vi "cRIO AI data2.vi"(0 "I":dbl, 1 "Input cluster":T1, 5 "error in (no error)":errorcluster, 6 "Chan 1":bool, 7 "Scale factor0":dbl, 9 "Scale factor1":dbl, 10 "Chan 2":bool, 11 "Scale factor2":dbl, 12 "Chan 3":bool, 13 "Scale factor3":dbl) -> (14 "Output data":dbl[](array[numeric]), 19 "error out":errorcluster)   [LabVIEW 2020]
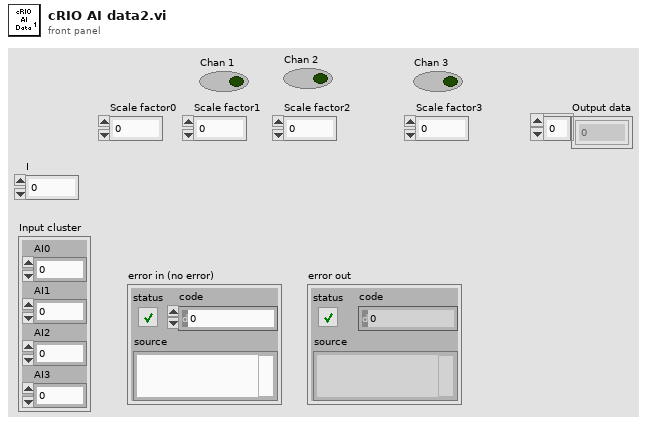
[diagram p1: front panel]
types:
  T1 = cluster{"AI0":dbl, "AI1":dbl, "AI2":dbl, "AI3":dbl}
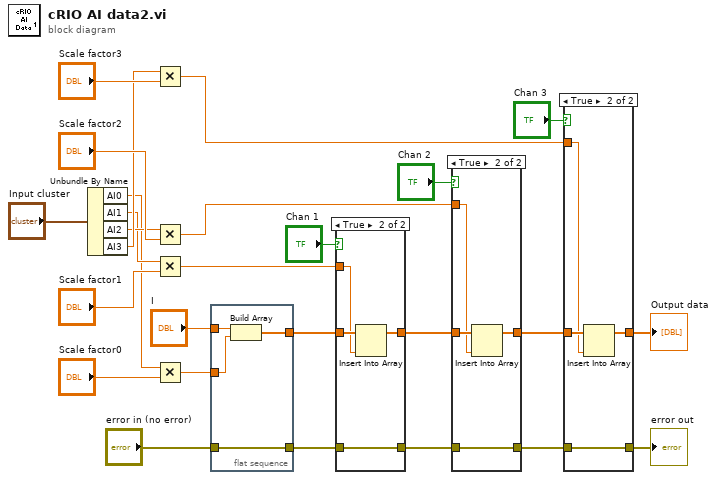
[diagram p0: block diagram]
diagram:
  n1 = Unbundle By Name("Input cluster") -> ("AI0"=w2:dbl, "AI1"=w3:dbl, "AI2"=w4:dbl, "AI3"=w5:dbl)
  n2 = Multiply(x=w5, y="Scale factor3") -> (x*y=w20:dbl)
  n3 = Multiply(x=w4, y="Scale factor2") -> (x*y=w19:dbl)
  n4 = Multiply(x=w3, y="Scale factor1") -> (x*y=w18:dbl)
  n5 = Multiply(x=w2, y="Scale factor0") -> (x*y=w17:dbl)
  n6 = flat-sequence {
    tunnel: "error in (no error)" -> [w30]
    tunnel: [w30] -> w13
    tunnel: w17 -> [w28]
    tunnel: [w29] -> w14
    tunnel: "I" -> [w27]
    frame #0 {
      n7 = Build Array(w27, w28) -> (w29:dbl[])
    }
  }
  n8 = case shown="True" "Chan 1" {
    tunnel: w13 -> [w31 w36]
    tunnel: [w31 w36] -> w10
    tunnel: w14 -> [w32 w35]
    tunnel: w18 -> [_ w34]
    tunnel: [w32 w33] -> w15
    frame False {
    }
    frame True {
      n9 = Insert Into Array(array=w35, new element=w34) -> (w33:dbl[])  [unwired: 1 in]
    }
  }
  n10 = case shown="True" "Chan 2" {
    tunnel: w10 -> [w37 w42]
    tunnel: [w37 w42] -> w11
    tunnel: w15 -> [w38 w41]
    tunnel: w19 -> [_ w40]
    tunnel: [w38 w39] -> w16
    frame False {
    }
    frame True {
      n11 = Insert Into Array(array=w41, new element=w40) -> (w39:dbl[])  [unwired: 1 in]
    }
  }
  n12 = case shown="True" "Chan 3" {
    tunnel: w11 -> [w43 w45]
    tunnel: w16 -> [w44 w48]
    tunnel: w20 -> [_ w47]
    tunnel: [w44 w46] -> w23
    tunnel: [w43 w45] -> w22
    frame False {
    }
    frame True {
      n13 = Insert Into Array(array=w48, new element=w47) -> (w46:dbl[])  [unwired: 1 in]
    }
  }
  "Output data" <- w23
  "error out" <- w22
